vi "FTW-Container-Initialize-IR.vi"(0 "Container":refnum<class "FTW-Container.lvclass">, 5 "Container IR":string, 11 "error in":errorcluster) -> (4 "Container out":refnum<class "FTW-Container.lvclass">, 15 "error out":errorcluster)   [LabVIEW 2012, in "FTW-Container.lvclass"]
uses:
  FTW-Container.lvclass
  FTW-Container.lvclass/FTW-Container.ctl
  <resource>/objmgr/DOMUserDefRef.rc
panel:
  # "Inputs"
  # "Outputs"
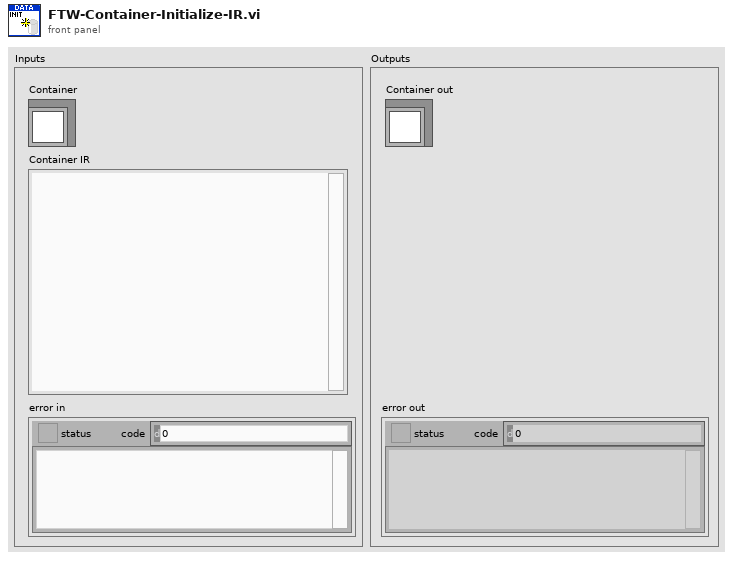
[diagram p1: front panel]
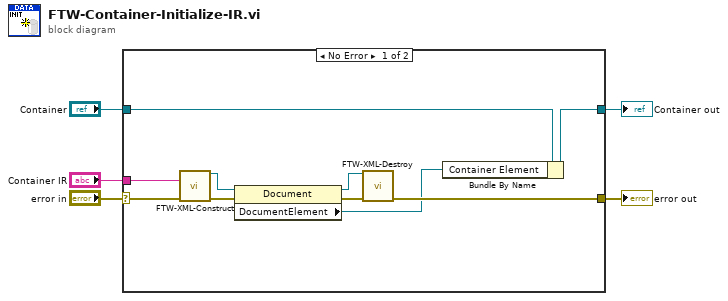
[diagram p0: block diagram]
diagram:
  n1 = case shown="No Error" "error in" {
    selector: "error in" -> [w9 w17]
    tunnel: [w7 w17] -> w5
    tunnel: [w14 w16] -> w1
    tunnel: "Container" -> [w15 w16]
    tunnel: "Container IR" -> [w8 _]
    frame No Error {
      n2 = call "FTW-XML-Construct.vi"("XML String"=w8, "error in"=w9) -> ("XML Document"=w13:refnum<k20>, "error out"=w12:errorcluster)  [unwired: 12 in]
      n3 = property class="Document"(reference=w13, error in=w12) -> (reference out=w11:refnum<k20>, error out=w10:errorcluster, "DocumentElement"=w6:refnum<k20>)
      n4 = call "FTW-XML-Destroy.vi"("XML Node"=w11, "error in"=w10) -> ("error out"=w7:errorcluster)  [unwired: 13 in]
      n5 = Bundle By Name(cluster=w15, "Container Element"=w6) -> (w14:refnum<class "FTW-Container.lvclass">)
    }
    frame Error {
    }
  }
  "error out" <- w5
  "Container out" <- w1
